vi "PipelineDuty.vi"(8 "error in (no error)":errorcluster, 10 "DataExchange":T1, 11 "GRMActor in":refnum<class "QuickNoteUI.lvclass">) -> (0 "error out":errorcluster, 2 "DataExchange Out":T1, 3 "GRMActor out":refnum<class "QuickNoteUI.lvclass">)   [LabVIEW 2020, in "QuickNoteUI.lvlib" / "QuickNoteUI.lvclass"]
uses:
  QuickNoteUI.lvclass
  Hardware Abstraction Layer/Component/Device/Device/DataExchange.ctl
  <vilib>/vision/Image Controls.llb/IMAQ Image.ctl
  QuickNoteUI.lvclass/QuickNoteUI.ctl
  Hardware Abstraction Layer/Component/GenericActor/GenericActor/GenericController.lvclass
  Interface/DataListener/DataListener.lvclass
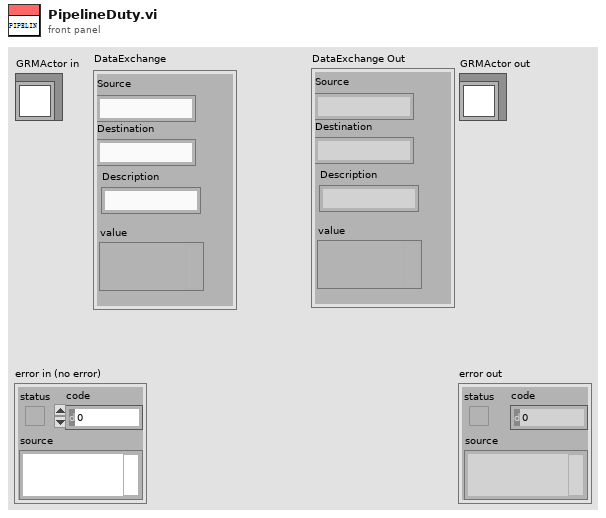
[diagram p1: front panel]
types:
  T1 = typedef "DataListener.lvclass/DataExchange.ctl" = cluster{"Source":string, "Destination":string, "Description":string, "value":variant}
  T2 = typedef "IMAQ Image.ctl" = refnum<image>
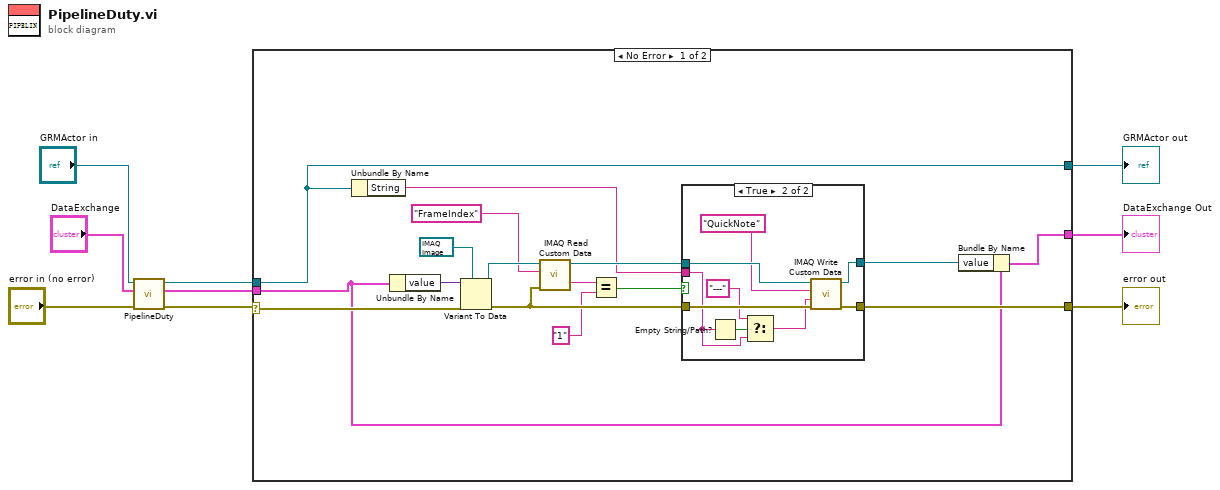
[diagram p0: block diagram]
diagram:
  n1 = call-parent "PipelineDuty.vi"("error in (no error)"="error in (no error)", "DataExchange"="DataExchange", "GRMActor in"="GRMActor in") -> ("error out"=w3:errorcluster, "DataExchange Out"=w5:T1, "GRMActor out"=w4:refnum<class "QuickNoteUI.lvclass">)  [unwired: 6 in]
  n2 = case shown="No Error" w3 {
    selector: w3 -> [w25 w39]
    tunnel: [w17 w39] -> w6
    tunnel: w5 -> [w12 w38]
    tunnel: w4 -> [w13 w37]
    tunnel: [w13 w37] -> w2
    tunnel: [w11 w38] -> w1
    frame No Error {
      n3 = Unbundle By Name(w13) -> ("String"=w15:string)
      n4 = Unbundle By Name(w12) -> ("value"=w24:variant)
      n5 = Variant To Data(error in=w25, type=T2 refnum ("Image"), Variant=w24) -> (data=w22:T2, error out=w20:errorcluster)
      n6 = call "IMAQ Read Custom Data"("error in (no error)"=w20, "Key"="FrameIndex", "Image"=w22) -> ("Custom Data Out"=w19:string, "Image (duplicate)"=w16:T2)  [unwired: 6 in, 1 out]
      n7 = Equal?(x=w19, y="1") -> (x = y?=w14:bool)
      n8 = case shown="True" w14 {
        tunnel: w20 -> [w27 w36]
        tunnel: [w27 w35] -> w17
        tunnel: w16 -> [w26 w34]
        tunnel: w15 -> [_ w30]
        tunnel: [w26 w32] -> w10
        frame False {
        }
        frame True {
          n9 = Empty String/Path?(string/path=w30) -> (empty?=w31:bool)
          n10 = Select(t="---", s=w31, f=w30) -> (s? t:f=w29:string)
          n11 = call "IMAQ Write Custom Data"("error in (no error)"=w36, "Custom Data In"=w29, "Key"="QuickNote", "Image"=w34) -> ("error out"=w35:errorcluster, "Image Out"=w32:T2)  [unwired: 6 in]
        }
      }
      n12 = Bundle By Name(cluster=w12, "value"=w10) -> (w11:T1)
    }
    frame Error {
    }
  }
  "error out" <- w6
  "GRMActor out" <- w2
  "DataExchange Out" <- w1
